vi "Launch Nested Actors.vi"(8 "error in (no error)":errorcluster, 11 "Elevator Controller in":refnum<class "Elevator Controller.lvclass">) -> (0 "error out":errorcluster, 3 "Elevator Controller out":refnum<class "Elevator Controller.lvclass">)   [LabVIEW 2019, in "Elevator Controller Actor.lvlib" / "Elevator Controller.lvclass"]
uses:
  Elevator Controller.lvclass
  C:/Program Files (x86)/National Instruments/LabVIEW 2019/vi.lib/ActorFramework/Actor/Actor.lvclass
  User Console Actor/User Console/User Console.lvclass
  Display Console/Display Console/Display Console.lvclass
  Sensor Interface Actor/Sensor Interface Actor/Sensor Interface.lvclass
  Configuration Database/Configuration Database Actor/Configuration Database.lvclass
  Elevator Controller.lvclass/Elevator Controller.ctl
  <vilib>/ActorFramework/Actor/Actor.lvclass
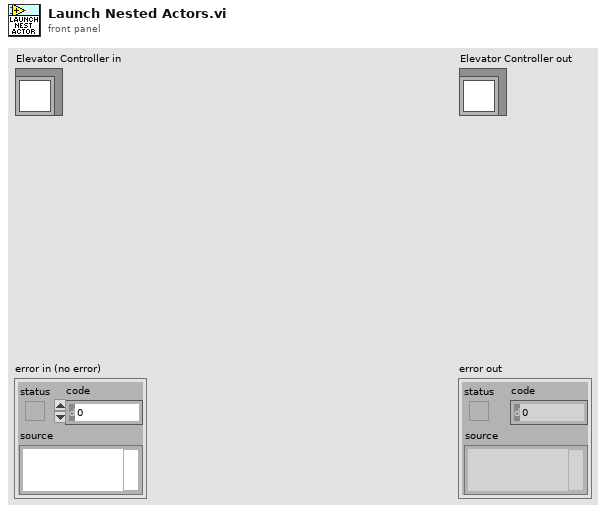
[diagram p1: front panel]
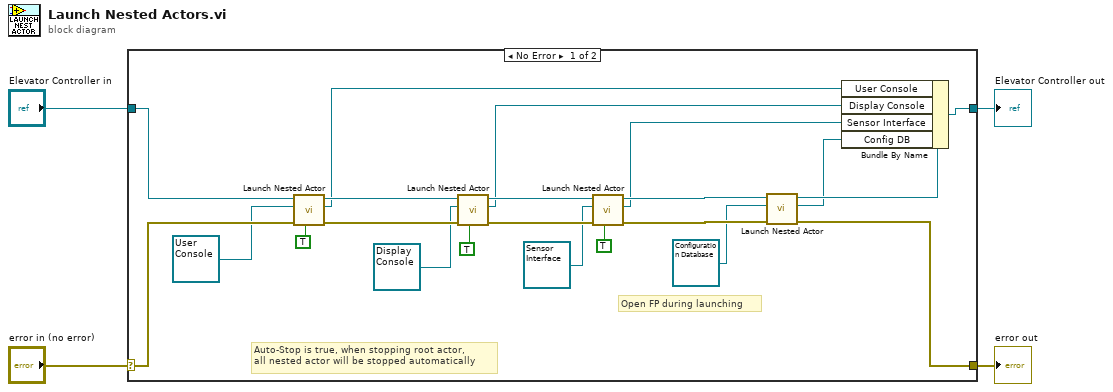
[diagram p0: block diagram]
diagram:
  n1 = case shown="No Error" "error in (no error)" {
    selector: "error in (no error)" -> [w24 w28]
    tunnel: [w12 w28] -> w3
    tunnel: [w26 w27] -> w1
    tunnel: "Elevator Controller in" -> [w16 w27]
    frame No Error {
      # "Auto-Stop is true, when stopping root actor, \nall nested actor will be stopped automatically"
      # "Open FP during launching"
      n2 = call <vilib>:"Launch Nested Actor.vi"("Open Actor Core front panel? (F)"=TRUE, "error in (no error)"=w24, "Nested Actor"=refnum<class "User Console.lvclass"> refnum ("User Console Actor.lvlib:User Console.lvclass"), "Caller Actor in"=w16) -> ("error out"=w23:errorcluster, "Nested Actor's Enqueuer"=w8:refnum<class "Message Enqueuer.lvclass">, "Caller Actor out"=w21:refnum<class "Elevator Controller.lvclass">)  [unwired: 5 in]
      n3 = call <vilib>:"Launch Nested Actor.vi"("Open Actor Core front panel? (F)"=TRUE, "error in (no error)"=w23, "Nested Actor"=refnum<class "Display Console.lvclass"> refnum ("Display Console Actor.lvlib:Display Console.lvclass"), "Caller Actor in"=w21) -> ("error out"=w22:errorcluster, "Nested Actor's Enqueuer"=w7:refnum<class "Message Enqueuer.lvclass">, "Caller Actor out"=w18:refnum<class "Elevator Controller.lvclass">)  [unwired: 5 in]
      n4 = call <vilib>:"Launch Nested Actor.vi"("Open Actor Core front panel? (F)"=TRUE, "error in (no error)"=w22, "Nested Actor"=refnum<class "Sensor Interface.lvclass"> refnum ("Sensor Interface Actor.lvlib:Display Console.lvclass"), "Caller Actor in"=w18) -> ("error out"=w19:errorcluster, "Nested Actor's Enqueuer"=w6:refnum<class "Message Enqueuer.lvclass">, "Caller Actor out"=w11:refnum<class "Elevator Controller.lvclass">)  [unwired: 5 in]
      n5 = call <vilib>:"Launch Nested Actor.vi"("error in (no error)"=w19, "Nested Actor"=refnum<class "Configuration Database.lvclass"> refnum ("Configuration Database Actor.lvlib:Configuration Database.lvclass"), "Caller Actor in"=w11) -> ("error out"=w12:errorcluster, "Nested Actor's Enqueuer"=w5:refnum<class "Message Enqueuer.lvclass">, "Caller Actor out"=w10:refnum<class "Elevator Controller.lvclass">)  [unwired: 6 in]
      n6 = Bundle By Name(cluster=w10, "User Console"=w8, "Display Console"=w7, "Sensor Interface"=w6, "Config DB"=w5) -> (w26:refnum<class "Elevator Controller.lvclass">)
    }
    frame Error {
    }
  }
  "error out" <- w3
  "Elevator Controller out" <- w1
